vi "Position YES NO Title String.vi"(8 "error in (no error)":errorcluster, 11 "String Ref":refnum<vi>) -> (0 "error out":errorcluster)   [LabVIEW 2014]
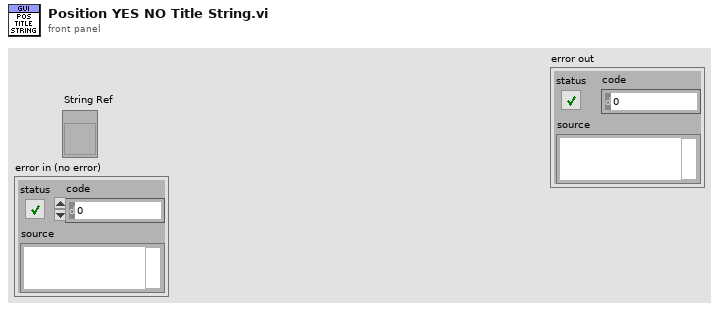
[diagram p1: front panel]
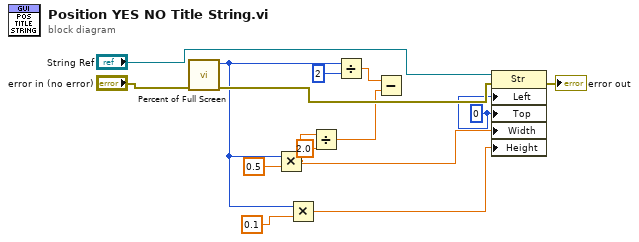
[diagram p0: block diagram]
diagram:
  w1 = 0 ("Position:Top")
  n1 = call "Percent of Full Screen.vi"("error in (no error)"="error in (no error)") -> ("error out"=w12:errorcluster, "Right"=w4:i16)  [unwired: 8 in, 1 out]
  n2 = Multiply(x=w4, y=0.5) -> (x*y=w8:dbl)
  n3 = Multiply(x=w4, y=0.1) -> (x*y=w2:dbl)
  n4 = Divide(x=w8, y=2.0) -> (x/y=w6:dbl)
  n5 = Divide(x=w4, y=i16 2) -> (x/y=w13:dbl)
  n6 = Subtract(x=w13, y=w6) -> ()  [unwired: 1 out]
  n7 = property class="Str"(reference="String Ref", error in=w12, "Left"=w1, "Top"=w1, "Width"=w8, "Height"=w2) -> (error out=→"error out":errorcluster)  [unwired: 1 out]
